vi "Eingabe Actual Point.vi"(8 "error in (no error)":errorcluster, 11 "TCP Network Connection in":refnum<k5>) -> (0 "error out":errorcluster, 2 "Actual Point":T1={"Punktnummer"="", "Transformation Point"={"dVal1"=0.0, "dVal2"=0.0, "dVal3"=0.0, "dStd1"=0.0001, "dStd2"=0.0001, "dStd3"=0.0001, "dCovar12"=0.0, "dCovar13"=0.0, "dCovar23"=0.0}}, 3 "TCP Network Connection out":refnum<k5>)   [LabVIEW 2017]
uses:
  AT901 API/Structures/Struct TransformationPointWithPointnumber.ctl
  AT901 API/Structures/Struct TransformationPoint.ctl
  AT901 API/TypeDefinitions/ES_MeasMode.ctl
  AT901 API/Structures/Struct StatisticModeParameter.ctl
  AT901 API/TypeDefinitions/ES_StatisticMode.ctl
panel:
  in  "Punktnummer":string
  out "dVal3":dbl
  out "dVal2":dbl
  out "dVal1":dbl
  in  "Messen":bool
  in  "stop":bool
  # "Bitte Punkt messen!"
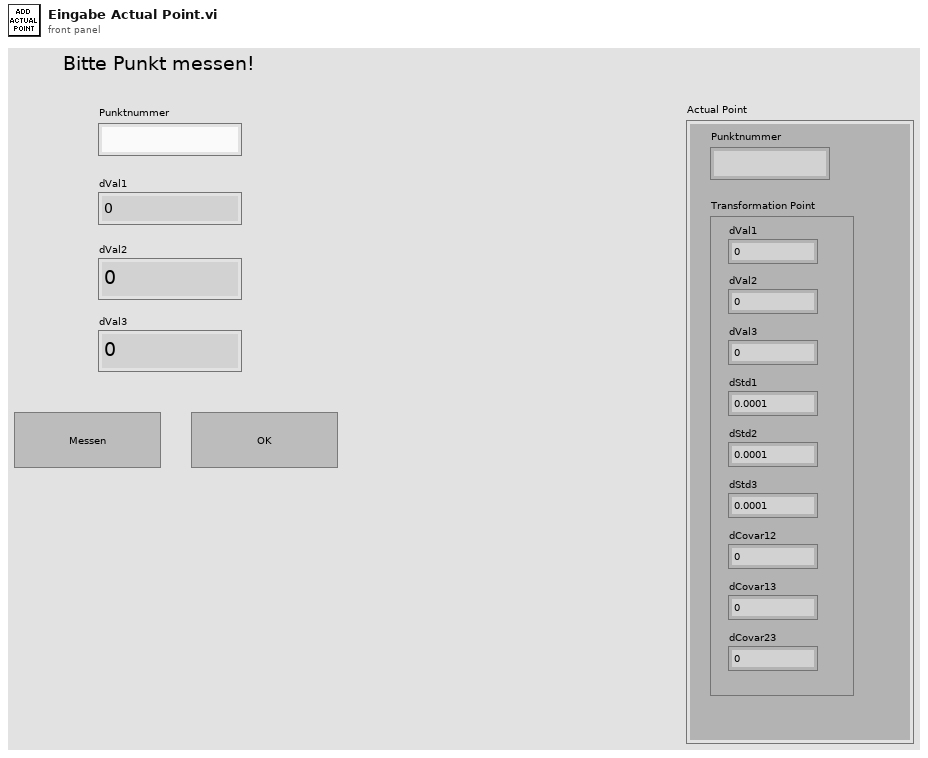
[diagram p1: front panel]
types:
  T1 = typedef "Struct TransformationPointWithPointnumber.ctl" = cluster{"Punktnummer":string, "Transformation Point":T2}
  T2 = typedef "Struct TransformationPoint.ctl" = cluster{"dVal1":dbl, "dVal2":dbl, "dVal3":dbl, "dStd1":dbl, "dStd2":dbl, "dStd3":dbl, "dCovar12":dbl, "dCovar13":dbl, "dCovar23":dbl}
  T3 = cluster{"Punktnummer":string, "Transformation Point":T2}
  T4 = typedef "Struct StatisticModeParameter.ctl" = cluster{"Statistic Mode Stationary":T5, "Statistic Mode Continuous":T5}
  T5 = typedef "ES_StatisticMode.ctl" = enum16{"ES_SM_Standard", "ES_SM_Extended"}
  T6 = typedef "ES_MeasMode.ctl" = enum32{"ES_MM_Stationary", "ES_MM_ContinuousTime", "ES_MM_ContinuousDistance", "ES_MM_Grid", "ES_MM_SphrereCenter", "ES_MM_CircleCenter", "ES_MM_6DStationary", "ES_MM_6DContinuousTime", "ES_MM_6DContinuousDistance", "ES_MM_6DGrid", "ES_MM_6DSphrereCenter", "ES_MM6DCircleCenter"}
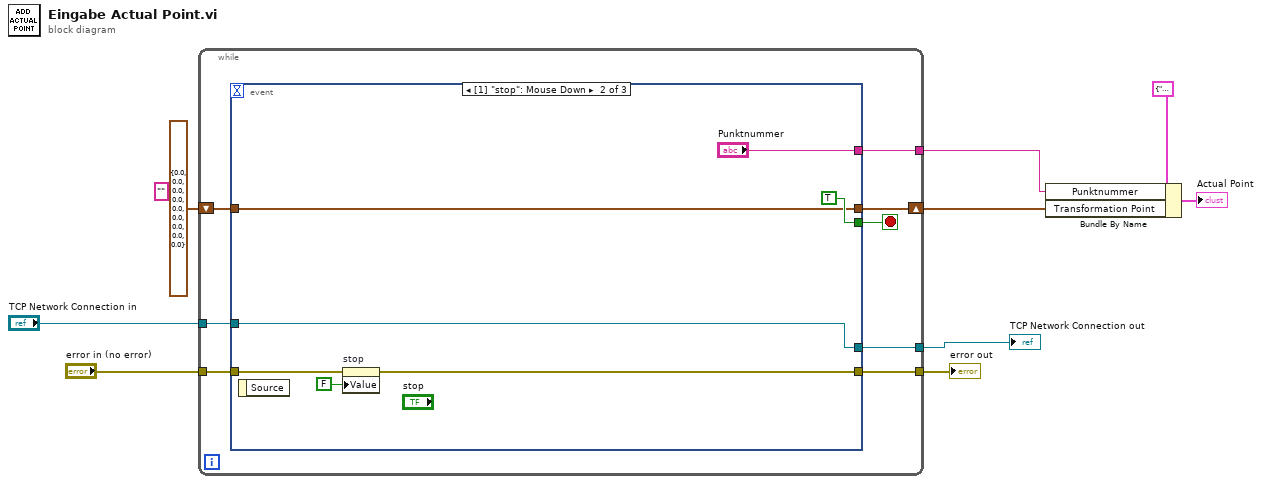
[diagram p0: block diagram]
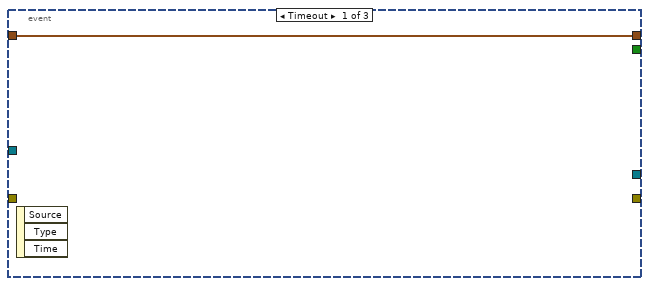
[diagram p2: hidden frame]
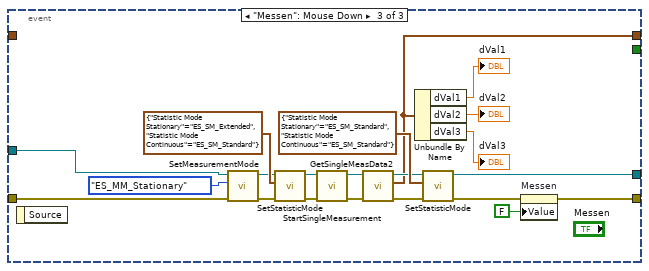
[diagram p3: hidden frame]
diagram:
  (unwired) "" ("Punktnummer")
  n1 = while {
    tunnel: "TCP Network Connection in" -> [w16]
    tunnel: "error in (no error)" -> [w15]
    tunnel: [w14] -> w7
    tunnel: [w13] -> w6
    shift-right: [w12] -> w2
    shift-left: T2 {"dVal1"=0.0, "dVal2"=0.0, "dVal3"=0.0, "dStd1"=0.0, "dStd2"=0.0, "dStd3"=0.0, "dCovar12"=0.0, "dCovar13"=0.0, "dCovar23"=0.0} ("Transformation Point") -> [w11]
    tunnel: [w10] -> w1
    stop <- w17 stop-if-true
    n2 = event shown="[1] \"stop\": Mouse Down" {
      selector: _ -> [_ _ _]
      dyn-events: _ -> [_ _ _]
      timeout: _ -> [_ _ _]
      tunnel: [_ TRUE _] -> w17
      tunnel: w16 -> [_ w23 w45]
      tunnel: w15 -> [_ w22 w44]
      tunnel: [_ w21 w42] -> w14
      tunnel: [_ w23 w33] -> w13
      tunnel: [w18 w20 w26] -> w12
      tunnel: w11 -> [w18 w20 _]
      tunnel: [_ "Punktnummer" _] -> w10
      event Timeout {
        n3 = event-data() -> ()  [unwired: 1 in, 3 out]
      }
      event "stop": Mouse Down {
        n4 = event-data() -> ()  [unwired: 1 in, 1 out]
        n5 = property on="stop" class="Bool (strict)"(error in=w22, "Value"=FALSE ("stop")) -> (error out=w21:errorcluster)  [unwired: 1 in, 1 out]
      }
      event "Messen": Mouse Down {
        n6 = event-data() -> ()  [unwired: 1 in, 1 out]
        n7 = call "SetMeasurementMode.vi"("error in (no error)"=w44, "ES_MeasMode"=ES_MeasMode."ES_MM_Stationary", "TCP Network Connection in"=w45) -> ("error out"=w30:errorcluster, "TCP Network Connection out"=w31:refnum<k5>)  [unwired: 5 in, 2 out]
        n8 = call "SetStatisticMode.vi"("error in (no error)"=w30, "Statistic Mode Params"=T4 {"Statistic Mode Stationary"=enum."ES_SM_Extended", "Statistic Mode Continuous"=enum."ES_SM_Standard"}, "TCP Network Connection in"=w31) -> ("error out"=w41:errorcluster, "TCP Network Connection out"=w40:refnum<k5>)  [unwired: 5 in, 2 out]
        n9 = call "StartSingleMeasurement.vi"("error in (no error)"=w41, "TCP Network Connection in"=w40) -> ("error out"=w37:errorcluster, "TCP Network Connection out"=w38:refnum<k5>)  [unwired: 7 in, 1 out]
        n10 = call "GetSingleMeasData2.vi"("error in (no error)"=w37, "TCP Network Connection in"=w38) -> ("error out"=w34:errorcluster, "Transformation Point"=w26:T2, "TCP Network Connection out"=w35:refnum<k5>)  [unwired: 6 in, 1 out]
        n11 = Unbundle By Name(w26) -> ("dVal1"=→"dVal1":dbl, "dVal2"=→"dVal2":dbl, "dVal3"=→"dVal3":dbl)
        n12 = call "SetStatisticMode.vi"("error in (no error)"=w34, "Statistic Mode Params"=T4 {"Statistic Mode Stationary"=enum."ES_SM_Standard", "Statistic Mode Continuous"=enum."ES_SM_Standard"}, "TCP Network Connection in"=w35) -> ("error out"=w32:errorcluster, "TCP Network Connection out"=w33:refnum<k5>)  [unwired: 5 in, 2 out]
        n13 = property on="Messen" class="Bool (strict)"(error in=w32, "Value"=FALSE ("Messen")) -> (error out=w42:errorcluster)  [unwired: 1 in, 1 out]
      }
    }
  }
  "error out" <- w7
  "TCP Network Connection out" <- w6
  n14 = Bundle By Name(cluster=T3 {"Punktnummer"="", "Transformation Point"={"dVal1"=0.0, "dVal2"=0.0, "dVal3"=0.0, "dStd1"=0.0, "dStd2"=0.0, "dStd3"=0.0, "dCovar12"=0.0, "dCovar13"=0.0, "dCovar23"=0.0}} ("Actual Point"), "Punktnummer"=w1, "Transformation Point"=w2) -> (→"Actual Point":T3)
